vi "Get Default Ref Phase.vi"(8 "error in (no error)":errorcluster, 11 "VISA resource name":refnum<visa-resource-name>) -> (0 "error out":errorcluster, 2 "Default Phase Value":dbl format="%.4f", 3 "VISA resource name out":refnum<visa-resource-name>)   [LabVIEW 2011, in "Fluke 5XXX Series Multicalibrators.lvlib"]
doc: "If two Calibrators are synchronized using 10 MHz IN/OUT, returns the power-up and reset default phase difference between the primary channel on the Calibrator and the sync pulse on the 10 MHz IN or OUT terminal.\n\nNote:\n\nThis VI is available only for instrument model 5520A."
uses:
  Fluke 5XXX Series Multicalibrators.lvlib
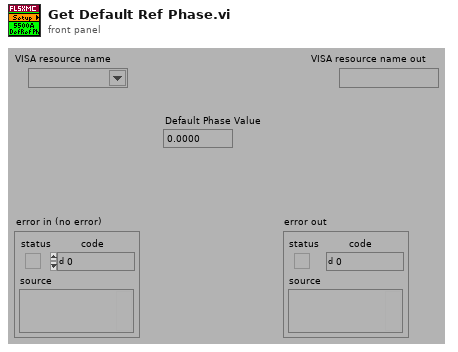
[diagram p1: front panel]
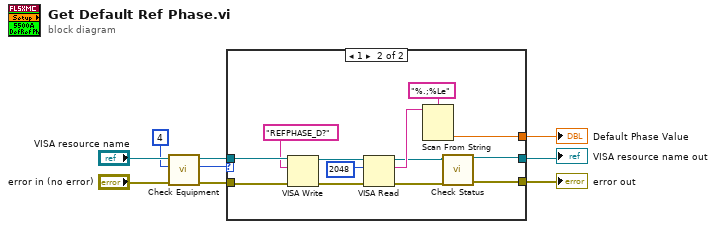
[diagram p0: block diagram]
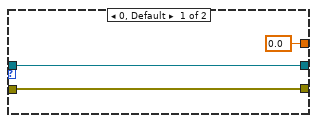
[diagram p2: hidden frame]
diagram:
  n1 = call "Check Equipment.vi"("error in (no error)"="error in (no error)", "Bit Mask"=4 ("Numeric"), "VISA resource name"="VISA resource name") -> ("error out"=w9:errorcluster, "Present?"=w8:u32, "VISA resource name out"=w7:refnum<visa-resource-name>)  [unwired: 6 in]
  n2 = case shown="1" w8 {
    tunnel: [w11 w24] -> w4
    tunnel: w9 -> [w12 w23]
    tunnel: w7 -> [w11 w22]
    tunnel: [w12 w25] -> w2
    tunnel: [0.0 w13] -> w3
    frame 0, Default {
    }
    frame 1 {
      n3 = VISA Write(VISA resource name=w22, write buffer="REFPHASE_D?", error in (no error)=w23) -> (VISA resource name out=w19:refnum<visa-resource-name>, error out=w18:errorcluster)  [unwired: 1 out]
      n4 = VISA Read(VISA resource name=w19, byte count=u32 2048 ("byte count (0)"), error in (no error)=w18) -> (VISA resource name out=w14:refnum<visa-resource-name>, read buffer=w15:string, error out=w16:errorcluster)  [unwired: 1 out]
      n5 = Scan From String(format string="%.;%Le", input string=w15) -> (output 1=w13:dbl)  [unwired: 3 in, 3 out]
      n6 = call "Check Status.vi"("VISA resource name"=w14, "error in (no error)"=w16) -> ("VISA resource name out"=w24:refnum<visa-resource-name>, "error out"=w25:errorcluster)  [unwired: 12 in]
    }
  }
  "Default Phase Value" <- w3
  "VISA resource name out" <- w4
  "error out" <- w2
